vi "32Bit_SignExtend Array.vi"(8 "Data In":u32[](array[numeric]), 9 "# data bits":i8) -> (0 "I32 data":i32[](array[numeric]) caption="I32 data (sign extended)")   [LabVIEW 2010, in "lib1299.lvlib"]
uses:
  lib1299.lvlib
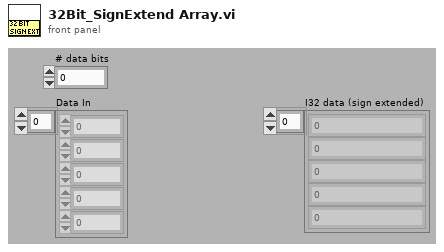
[diagram p1: front panel]
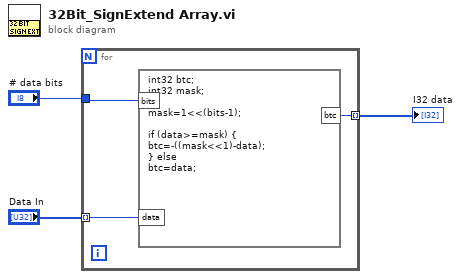
[diagram p0: block diagram]
diagram:
  n1 = for {
    tunnel: "Data In" -> [w6] mode=indexing
    tunnel: "# data bits" -> [w5]
    tunnel: [w4] -> w3 mode=indexing
    n2 = formula code="int32 btc;\nint32 mask;\n\nmask=1<<(bits-1);\n\nif (data>=mask) {\nbtc=-((mask<<1)-data);\n} else\nbtc=data;"("bits"=w5, "data"=w6) -> ("btc"=w4:i32)
  }
  "I32 data" <- w3
